vi "U16s to Bytes.vi"(11 "registers":u16[](array[numeric])) -> (2 "bytes":u8[](array[numeric]), 3 "count":u8)   [LabVIEW 2020, in "SubVIs.lvlib"]
doc: "Converts words into bytes."
uses:
  <vilib>/Modbus/subvis/SubVIs.lvlib
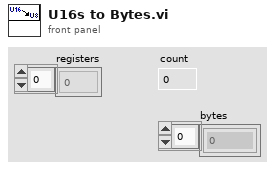
[diagram p1: front panel]
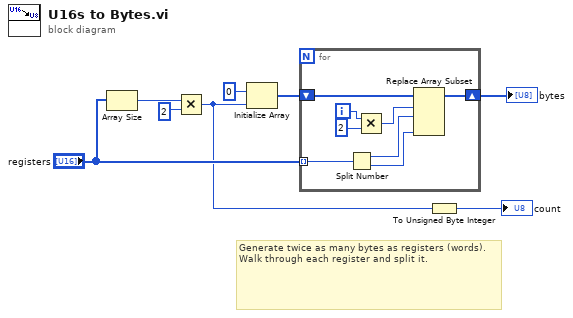
[diagram p0: block diagram]
diagram:
  # "Generate twice as many bytes as registers (words). Walk through each register and split it."
  n1 = Array Size(array="registers") -> (size(s)=w7:i32)
  n2 = Multiply(x=w7, y=2) -> (x*y=w2:i32)
  n3 = Initialize Array(u8 0, w2) -> (w4:u8[])
  n4 = for {
    tunnel: "registers" -> [w16] mode=indexing
    shift-right: [w14] -> w3
    shift-left: w4 -> [w15]
    i -> [w11]
    n5 = Split Number(x=w16) -> (hi(x)=w12:u8, lo(x)=w13:u8)
    n6 = Multiply(x=w11, y=2) -> (x*y=w9:i32)
    n7 = Replace Array Subset(array=w15, new element #1=w12, index #1=w9, new element #2=w13) -> (w14:u8[])  [unwired: 1 in]
  }
  "bytes" <- w3
  n8 = To Unsigned Byte Integer(number=w2) -> (unsigned 8bit integer=→"count":u8)
